vi "InhibitPEM100.vi"() -> ()   [LabVIEW 2011]
panel:
  out "Wavelength":dbl caption="(nm)" format="%.2g"
  out "error out":errorcluster
  in  "Inhibit":bool
  in  "VISA session":refnum<visa-resource-name>
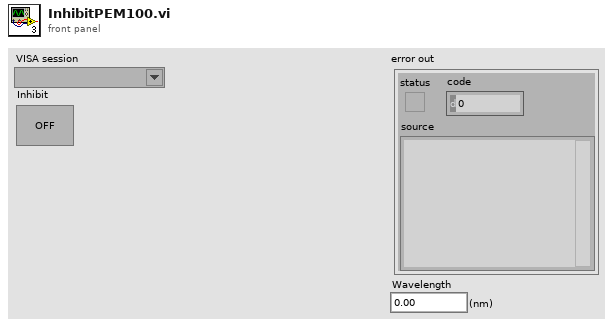
[diagram p1: front panel]
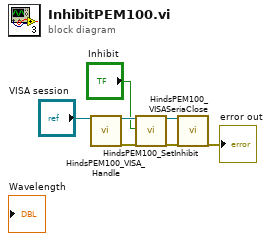
[diagram p0: block diagram]
diagram:
  n1 = call "HindsPEM100_VISA_Handle.vi"("VISA session"="VISA session") -> ("VISA refnum out"=w5:refnum<visa-resource-name>, "error out"=w3:errorcluster)  [unwired: 17 in]
  n2 = call "HindsPEM100_SetInhibit.vi"("VISA refnum in"=w5, "Inhibit"="Inhibit", "error in (no error)"=w3) -> ("VISA refnum out"=w4:refnum<visa-resource-name>, "error out"=w2:errorcluster)  [unwired: 15 in]
  n3 = call "HindsPEM100_VISASeriaClose.vi"("VISA session (for class)"=w4, "error in (no error)"=w2) -> ("error out"=→"error out":errorcluster)  [unwired: 17 in]
